vi "DigitalInputStart.vi"(0 "Device Info":T1={"Serial Number"=-1, "Channel"=0, "Port"=0}, 1 "Input Mode":i32(ring)=1 items=["INPUT_MODE_NPN"=1, "INPUT_MODE_PNP"=2], 2 "Power Supply":i32(ring)=2 items=["POWER_SUPPLY_OFF"=1, "POWER_SUPPLY_12V"=2, "POWER_SUPPLY_24V"=3], 5 "IsHubPort":bool, 11 "error in (no error)":errorcluster, 12 "Connection":u16(ring) items=["No Preference", "Remote", "Local"], 13 "Timeout (mSec)":i32=5000) -> (4 "Phidget ID":u64, 6 "Serial Number Return":i32, 10 "Attached?":bool, 15 "error out":errorcluster)   [LabVIEW 2020, in "Phidget Digital Input.lvlib"]
doc: "${DigitalInput:StartHeader}"
uses:
  <instrlib>/Phidgets/Phidget Digital Input/Phidget Digital Input.lvlib
  <instrlib>/Phidgets/Phidget Common/Phidget Common.lvlib
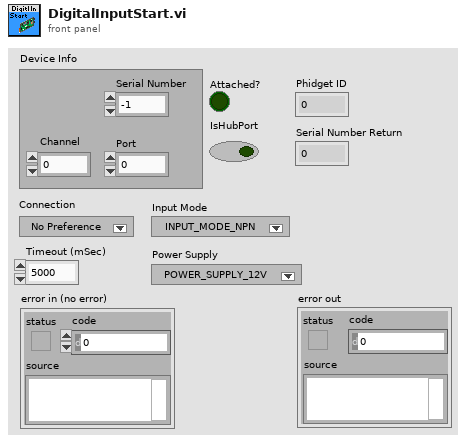
[diagram p1: front panel]
types:
  T1 = cluster{"Serial Number":i32, "Channel":i32, "Port":i32}
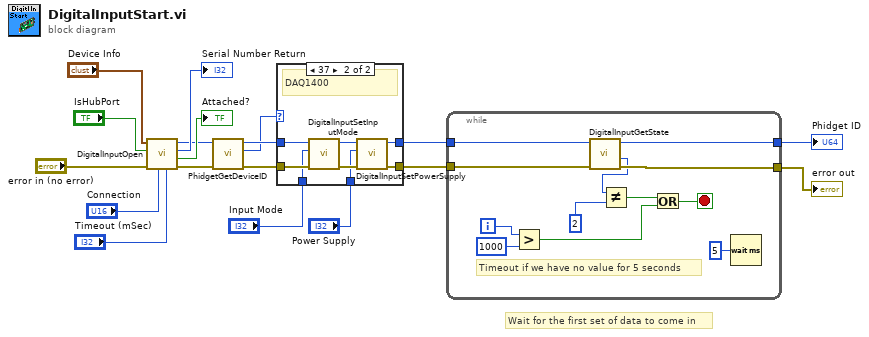
[diagram p0: block diagram]
diagram:
  # "Wait for the first set of data to come in"
  n1 = call <instrlib>:"DigitalInputOpen.vi"("Timeout (mSec)"="Timeout (mSec)", "Connection"="Connection", "error in"="error in (no error)", "IsHubPort"="IsHubPort", "Device Info"="Device Info") -> ("error out"=w8:errorcluster, "Attached?"=→"Attached?":bool, "Serial Number Return"=→"Serial Number Return":i32, "Phidget ID"=w9:u64)  [unwired: 3 in]
  n2 = call <instrlib>:"PhidgetGetDeviceID.vi"("error in (no error)"=w8, "Device In"=w9) -> ("error out"=w6:errorcluster, "Devie IDs"=w5:u32, "Device Out"=w7:u64)  [unwired: 6 in]
  n3 = case shown="37" w5 {
    tunnel: w7 -> [w20 w27]
    tunnel: w6 -> [w19 w28]
    tunnel: [w20 w23] -> w4
    tunnel: [w19 w24] -> w3
    tunnel: "Input Mode" -> [_ w22]
    tunnel: "Power Supply" -> [_ w21]
    frame 0, Default {
    }
    frame 55 {
      # "DAQ1400"
      n4 = call <instrlib>:"DigitalInputSetInputMode.vi"("error in (no error)"=w28, "Input Mode"=w22, "Device In"=w27) -> ("error out"=w25:errorcluster, "Device Out"=w26:u64)  [unwired: 6 in]
      n5 = call <instrlib>:"DigitalInputSetPowerSupply.vi"("error in (no error)"=w25, "Power Supply"=w21, "Device In"=w26) -> ("error out"=w24:errorcluster, "Device Out"=w23:u64)  [unwired: 6 in]
    }
  }
  n6 = while {
    tunnel: w4 -> [w38]
    tunnel: w3 -> [w37]
    tunnel: [w35] -> w10
    tunnel: [w36] -> w11
    i -> [w33]
    stop <- w30 stop-if-true
    # "Timeout if we have no value for 5 seconds"
    n7 = Greater?(x=w33, y=1000) -> (0:w31:bool)
    n8 = call <instrlib>:"DigitalInputGetState.vi"("error in (no error)"=w37, "Device In"=w38) -> ("error out"=w36:errorcluster, "State (Numeric)"=w29:i32, "Device Out"=w35:u64)  [unwired: 5 in, 1 out]
    n9 = Not Equal?(x=w29, y=2) -> (x != y?=w32:bool)
    n10 = Or(x=w32, y=w31) -> (x .or. y?=w30:bool)
    n11 = Wait (ms)(milliseconds to wait=u32 5) -> ()  [unwired: 1 out]
  }
  "error out" <- w11
  "Phidget ID" <- w10
